vi "进度条v1.2.1.vi"() -> ()   [LabVIEW 2018]
panel:
  out "进度显示":dbl format="%#.2f%%"
  out "水平刻度条":dbl(slide) scale=0.0..100.0
  # "正在识别，请等待！"
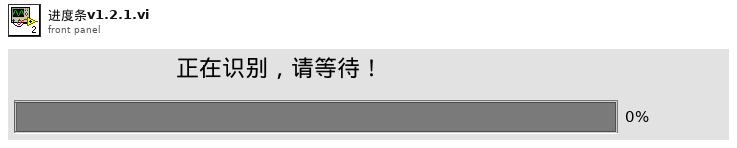
[diagram p1: front panel]
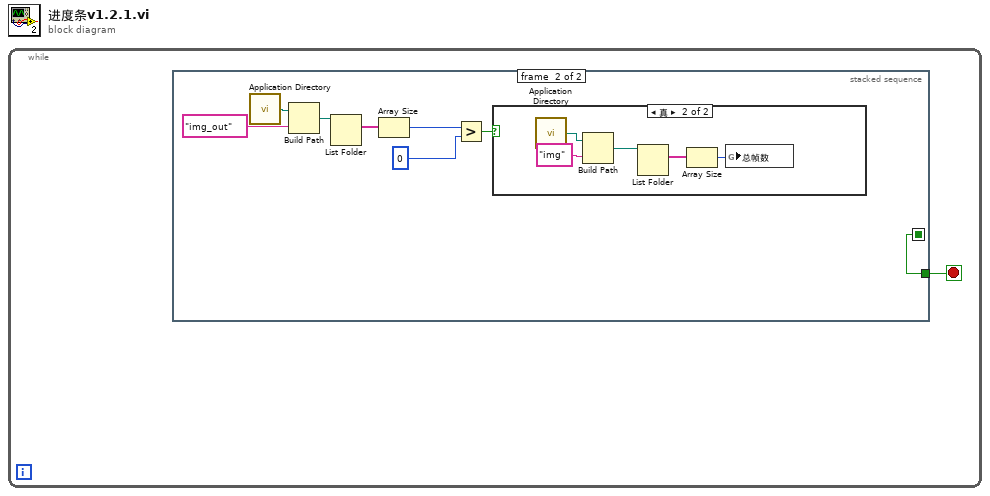
[diagram p0: block diagram]
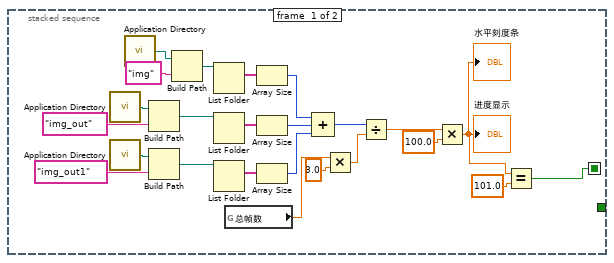
[diagram p2: hidden frame]
diagram:
  n1 = while {
    stop <- w1 stop-if-true
    n2 = stacked-sequence {
      seq-local: [w2 _] -> [_ w33]
      tunnel: [_ w33] -> w1
      frame #0 {
        n3 = call <vilib>:"Application Directory.vi"() -> ("Application Directory"=w18:path)
        n4 = call <vilib>:"Application Directory.vi"() -> ("Application Directory"=w19:path)
        n5 = call <vilib>:"Application Directory.vi"() -> ("Application Directory"=w6:path)
        n6 = Build Path(base path=w18, name or relative path="img_out" ("名称或相对路径")) -> (appended path=w17:path)
        n7 = Build Path(base path=w19, name or relative path="img_out1" ("名称或相对路径")) -> (appended path=w20:path)
        n8 = Build Path(base path=w6, name or relative path="img" ("名称或相对路径")) -> (appended path=w7:path)
        n9 = List Folder(path=w7) -> (filenames=w5:string[])  [unwired: 3 in, 3 out]
        n10 = List Folder(path=w17) -> (filenames=w21:string[])  [unwired: 3 in, 3 out]
        n11 = List Folder(path=w20) -> (filenames=w22:string[])  [unwired: 3 in, 3 out]
        n12 = global read "全局变量.vi" "总帧数"() -> (w3:dbl)
        n13 = Array Size(array=w5) -> (size(s)=w4:i32)
        n14 = Array Size(array=w21) -> (size(s)=w23:i32)
        n15 = Array Size(array=w22) -> (size(s)=w24:i32)
        n16 = Compound Arithmetic op=ADD(w4, w23, w24) -> (w14:i32)
        n17 = Multiply(x=w3, y=3.0) -> (x*y=w13:dbl)
        n18 = Divide(x=w14, y=w13) -> (x/y=w11:dbl)
        n19 = Multiply(x=w11, y=100.0) -> (x*y=w10:dbl)
        "水平刻度条" <- w10
        "进度显示" <- w10
        n20 = Equal?(x=w10, y=101.0) -> (x = y?=w2:bool)
      }
      frame #1 {
        n21 = call <vilib>:"Application Directory.vi"() -> ("Application Directory"=w30:path)
        n22 = Build Path(base path=w30, name or relative path="img_out" ("名称或相对路径")) -> (appended path=w31:path)
        n23 = List Folder(path=w31) -> (filenames=w29:string[])  [unwired: 3 in, 3 out]
        n24 = Array Size(array=w29) -> (size(s)=w28:i32)
        n25 = Greater?(x=w28, y=0) -> (0:w26:bool)
        n26 = case shown="真" w26 {
          frame False {
          }
          frame True {
            n27 = call <vilib>:"Application Directory.vi"() -> ("Application Directory"=w37:path)
            n28 = Build Path(base path=w37, name or relative path="img" ("名称或相对路径")) -> (appended path=w36:path)
            n29 = List Folder(path=w36) -> (filenames=w38:string[])  [unwired: 3 in, 3 out]
            n30 = Array Size(array=w38) -> (size(s)=w34:i32)
            n31 = global write "全局变量.vi" "总帧数"(w34) -> ()
          }
        }
      }
    }
  }
